vi "UpdateCallLibraryNodePaths.vi"   [LabVIEW 2020]
uses:
  <vilib>/Utility/traverseref.llb/TRef TravTarget.ctl
  <vilib>/Utility/traverseref.llb/VI Scripting - Traverse.lvlib
types:
  T1 = typedef "TRef TravTarget.ctl" = enum16{"FP", "BD", "Other"}
  T2 = enum32{"Invalid", "Standard", "Closed", "Hidden", "Minimized", "Maximized"}
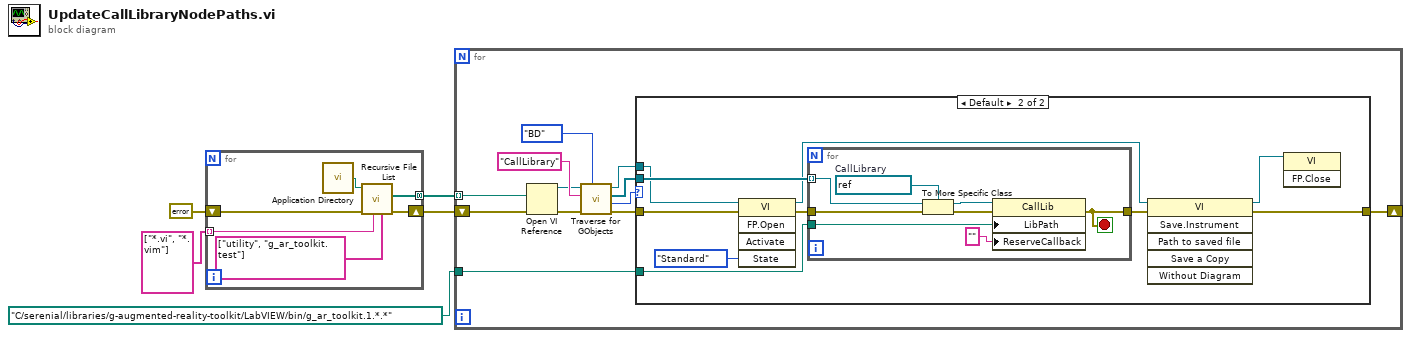
[diagram p0: block diagram]
diagram:
  n1 = for {
    tunnel: string[] ["*.vi", "*.vim"] ("pattern") -> [w11] mode=indexing
    tunnel: [w10] -> w1 mode=concatenating
    shift-right: [w8] -> w4
    shift-left: errorcluster {"status"=FALSE, "code"=0, "source"=""} ("error constant") -> [w7]
    n2 = call <vilib>:"Application Directory.vi"() -> ("Application Directory"=w9:path)
    n3 = call <vilib>:"Recursive File List.vi"("Folders to Exclude"=string[] ["utility", "g_ar_toolkit.test"], "pattern"=w11, "error in (no error)"=w7, "Folder Path"=w9) -> ("error out"=w8:errorcluster, "All Files in Dir"=w10:path[])  [unwired: 3 in, 3 out]
  }
  n4 = for {
    tunnel: w1 -> [w20] mode=indexing
    shift-right: [w23] -> _
    shift-left: w4 -> [w22]
    tunnel: path "C:/serenial/libraries/g-augmented-reality-toolkit/LabVIEW/bin/g_ar_toolkit.1.*.*" ("Library Path") -> [w21]
    n5 = Open VI Reference(vi path=w20, error in (no error)=w22) -> (vi reference=w12:refnum<vi>, error out=w13:errorcluster)  [unwired: 4 in]
    n6 = call <vilib>:"Traverse for GObjects.vi"("Traverse Target"=TRef_TravTarget."BD", "error in (no error)"=w13, "Class Name"="CallLibrary", "VI Refnum"=w12) -> ("error out"=w16:errorcluster, "# of Refs"=w14:i32, "References"=w17:refnum<vi>[], "dup VI Refnum"=w15:refnum<vi>)  [unwired: 4 in]
    n7 = case shown="Default" w14 {
      tunnel: w17 -> [_ w34]
      tunnel: w16 -> [w24 w30]
      tunnel: w15 -> [_ w26]
      tunnel: [w24 w33] -> w23
      tunnel: w21 -> [_ w31]
      frame 0 {
      }
      frame Default {
        n8 = invoke class="VI" method="FP.Open"(reference=w26, error in=w30, "State"=T2."Standard") -> (reference out=w25:refnum<vi>, error out=w29:errorcluster)  [unwired: 2 in, 3 out]
        n9 = for {
          tunnel: w34 -> [w42] mode=indexing
          tunnel: w29 -> [w40]
          tunnel: [w38] -> w32
          tunnel: w31 -> [w36]
          stop <- w38 stop-if-true
          w37 = refnum<vi> refnum  # CallLibrary
          n10 = To More Specific Class(target class=w37, reference=w42, error in=w40) -> (specific class reference=w41:refnum<vi>, error out=w39:errorcluster)
          n11 = property class="CallLib"(reference=w41, error in=w39, "LibPath"=w36, "ReserveCallback"="" ("Reserve Callback")) -> (error out=w38:errorcluster)  [unwired: 1 out]
        }
        n12 = invoke class="VI" method="Save.Instrument"(reference=w25, error in=w32) -> (reference out=w27:refnum<vi>, error out=w33:errorcluster)  [unwired: 4 in, 4 out]
        n13 = invoke class="VI" method="FP.Close"(reference=w27) -> ()  [unwired: 2 in, 3 out]
      }
    }
  }
